vi "test.vi"() -> ()   [LabVIEW 2019]
panel:
  out "Array 2":dbl[](array[numeric])
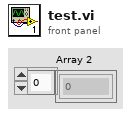
[diagram p1: front panel]
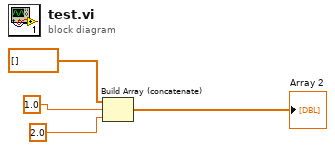
[diagram p0: block diagram]
diagram:
  n1 = Build Array (concatenate)(dbl[] [], 1.0, 2.0) -> (→"Array 2":dbl[])
